vi "PascoButtonArrayToInt.vi"(11 "Button Array":bool[](array[boolean])) -> (3 "s? t:f":i32)   [LabVIEW 2012]
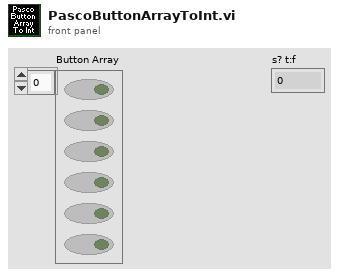
[diagram p1: front panel]
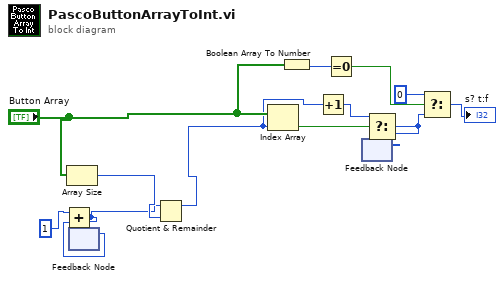
[diagram p0: block diagram]
diagram:
  n1 = Array Size(array="Button Array") -> (size(s)=w14:i32)
  n2 = feedback #1() -> (w3:i32)  [unwired: 1 in]
  n3 = Add(x=1 ("Iterations"), y=w3) -> (x+y=w2:i32)
  n4 = feedback-in #1(w2) -> ()
  n5 = Quotient & Remainder(x=w2, y=w14) -> (x-y*floor(x/y)=w4:i32)  [unwired: 1 out]
  n6 = Index Array(array="Button Array", index=w4) -> (element=w13:bool)
  n7 = Boolean Array To Number(Boolean array="Button Array") -> (number=w10:u32)
  n8 = Increment(x=w4) -> (x+1=w5:i32)
  n9 = Equal To 0?(x=w10) -> (x = 0?=w9:bool)
  n10 = feedback #2() -> (w12:i32)  [unwired: 1 in]
  n11 = Select(t=w5, s=w13, f=w12) -> (s? t:f=w7:i32)
  n12 = feedback-in #2(w7) -> ()
  n13 = Select(t=0, s=w9, f=w7) -> (s? t:f=→"s? t:f":i32)
